vi "Launch Blocks UI.vi"(8 "error in (no error)":errorcluster) -> (0 "error out":errorcluster)   [LabVIEW 2022 SP3, in "FlexBlocks Support.lvlib"]
uses:
  FlexBlocks Support.lvlib
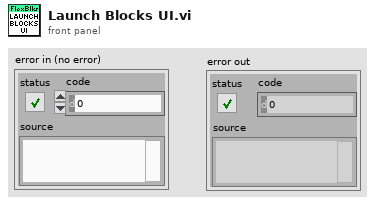
[diagram p1: front panel]
types:
  T1 = enum32{"Invalid", "Standard", "Closed", "Hidden", "Minimized", "Maximized"}
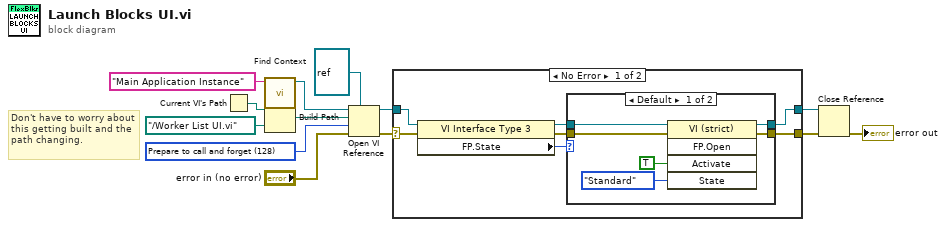
[diagram p0: block diagram]
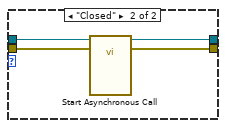
[diagram p2: hidden frame]
diagram:
  w13 = 128 items=["Record modifications"=1, "Open templates for editing"=2, "Prompt user to save"=4, "Prepare for reentrant run"=8, "Prompt to find missing subVIs"=16, "Hide loading dialog box"=32, "Enable simultaneous calls"=64, "Prepare to call and forget"=128, "Simultaneous call and forget"=192, "Prepare to call and collect"=256, "Simultaneous call and collect"=320]
  # "Don't have to worry about this getting built and the path changing."
  n1 = Current VI's Path() -> (path=w5:path)
  n2 = call "Find Context.vi"("Name"="Main Application Instance") -> ("App"=w11:refnum<vi>)  [unwired: 9 in, 1 out]
  n3 = Build Path(base path=w5, name or relative path=path "../Worker List UI.vi") -> (appended path=w2:path)
  n4 = Open VI Reference(type specifier VI Refnum (for type only)=refnum<vi> refnum, application reference (local)=w11, vi path=w2, options=w13, error in (no error)="error in (no error)") -> (vi reference=w8:refnum<vi>, error out=w9:errorcluster)  [unwired: 1 in]
  n5 = case shown="No Error" w9 {
    selector: w9 -> [w18 w32]
    tunnel: w8 -> [w20 w31]
    tunnel: [w15 w31] -> w7
    tunnel: [w14 w32] -> w6
    frame No Error {
      n6 = property class="VI Interface Type 3"(reference=w20, error in=w18) -> (reference out=w19:refnum<vi>, error out=w17:errorcluster, "FP.State"=w16:T1)
      n7 = case shown="Default" w16 {
        tunnel: w19 -> [w22 w30]
        tunnel: w17 -> [w21 w29]
        tunnel: [w24 w28] -> w15
        tunnel: [w23 w27] -> w14
        frame Default {
          n8 = invoke class="VI (strict)" method="FP.Open"(reference=w22, error in=w21, "Activate"=TRUE ("Activate?"), "State"=T1."Standard") -> (reference out=w24:refnum<vi>, error out=w23:errorcluster)  [unwired: 1 in, 3 out]
        }
        frame "Closed" {
          n9 = call-by-ref "Start Asynchronous Call"(reference=w30, error in=w29) -> (reference out=w28:refnum<vi>, error out=w27:errorcluster)  [unwired: 12 in]
        }
      }
    }
    frame Error {
    }
  }
  n10 = Close Reference(reference=w7, error in (no error)=w6) -> (error out=→"error out":errorcluster)
